vi "Read Key.vi"(8 "Error In":errorcluster, 11 "Known Host In":refnum<class "Known Host.lvclass">) -> (0 "Error Out":errorcluster, 2 "Key":u8[](array[numeric]), 3 "Known Host Out":refnum<class "Known Host.lvclass">)   [LabVIEW 2018, in "Toolkit.lvlib" / "Known Host.lvclass"]
uses:
  Known Host.lvclass
  Known Host.lvclass/Known Host.ctl
  SSH/SSH.lvclass/SSH.ctl
  Toolkit.lvlib
  SSH/SSH.lvclass
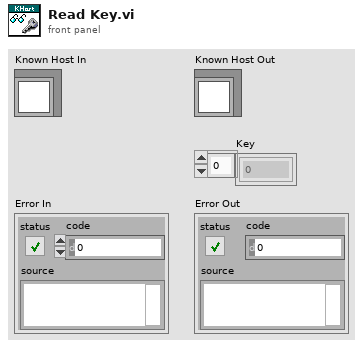
[diagram p1: front panel]
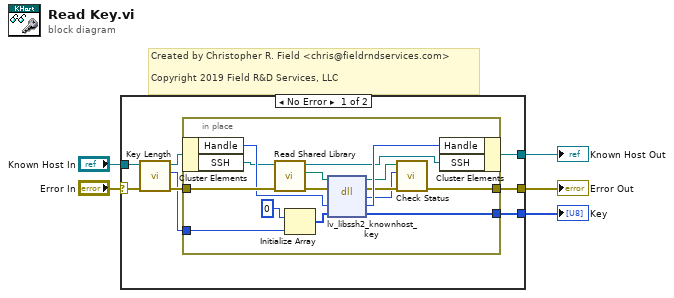
[diagram p0: block diagram]
diagram:
  # "Created by Christopher R. Field <chris@fieldrndservices.com>\n\nCopyright 2019 Field R&D Services, LLC"
  n1 = case shown="No Error" "Error In" {
    selector: "Error In" -> [w12 w30]
    tunnel: [w13 w30] -> w4
    tunnel: "Known Host In" -> [w10 w29]
    tunnel: [w7 w29] -> w2
    tunnel: [w6 _] -> w1
    frame No Error {
      n2 = call "Key Length.vi"("Error In"=w12, "Known Host In"=w10) -> ("Error Out"=w11:errorcluster, "Length"=w8:u64, "Known Host Out"=w9:refnum<class "Known Host.lvclass">)  [unwired: 7 in]
      n3 = in-place {
        in-place-border: w11 -> [w28]
        in-place-border: [w25] -> w13
        in-place-border: w8 -> [w21]
        in-place-border: [w18] -> w6
        n4 = in-place-cluster #1(w9) -> ("Handle"=w19:u64, "SSH"=w16:refnum<class "SSH.lvclass">)
        n5 = call "Read Shared Library.vi"("Error In"=w28, "SSH In"=w16) -> ("Error Out"=w17:errorcluster, "libssh2lv Shared Library"=w15:path, "SSH Out"=w14:refnum<class "SSH.lvclass">)  [unwired: 7 in]
        n6 = Initialize Array(u8 0, w21) -> (w20:u8[])
        n7 = dll-call lib="lv-libssh2.*" fn="lv_libssh2_knownhost_key"(path in=w15, error in=w17, "handle"=w19, "buffer"=w20) -> (path out=w24:path, error out=w26:errorcluster, "status"=w23:i32, "handle"=w27:u64, "buffer"=w18:u8[])  [unwired: 1 in]
        n8 = call "Check Status.vi"("Error In"=w26, "Status"=w23, "lv-libssh2 Shared Library In"=w24) -> ("Error Out"=w25:errorcluster)  [unwired: 7 in, 1 out]
        n9 = in-place-cluster #1("Handle"=w27, "SSH"=w14) -> (w7:refnum<class "Known Host.lvclass">)
      }
    }
    frame Error {
    }
  }
  "Error Out" <- w4
  "Known Host Out" <- w2
  "Key" <- w1
